vi "second_order_system_mathscript.calculate.vi"() -> ()   [LabVIEW 2015]
uses:
  <vilib>/addons/Control Design/_Model Construction/Model Typedefs.llb/CD General Elements.ctl
  <vilib>/addons/Control Design/_Model Construction/NI_LinSys_Model Typedefs.lvlib
  <vilib>/addons/Control Design/_Model Construction/Model Typedefs.llb/CD Transfer Function Model (SISO).ctl
  <vilib>/addons/Control Design/_Model Construction/Model Typedefs.llb/CD Transfer Function Model (MIMO).ctl
panel:
  in  "Step Time (s)":dbl=3.0
  in  "Gain":dbl=110000.0
  out "SysDis":T1={"properties"={"Model name"="System Model", "Input names"=["u0"], "Output names"=["y0"], "Input Delays"=[0.0], "Output Delays"=[0.0], "Sampling Time"=2e-05, "Notes"=""}, "transfer function(s)"=[[{"Numerator"=[2.19982359548343e-05, 2.1999115901172317e-05], "Denominator"=[0.9998800071997122, -1.9998777573351285, 1.0], "delay"=0.0}]]} caption="TF object" {"transfer function(s)"."delay" format="%.4f"; "transfer function(s)"."Denominator" format="%#_9e"; "transfer function(s)"."Numerator" format="%#_9e"; "properties"."Sampling Time" format="%#.6p"; "properties"."Output Delays" format="%.4f"; "properties"."Input Delays" format="%.4f"}
  in  "Ts":dbl=2e-05
  in  "NaturalFreq (r/s)":dbl=75.0
  in  "DampingRatio":dbl=0.04
  # "For the step response plot"
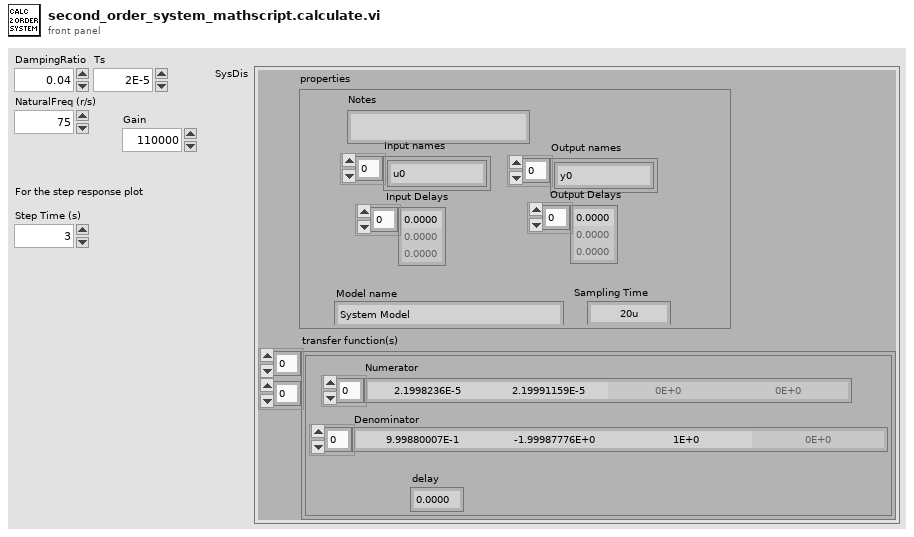
[diagram p1: front panel]
types:
  T1 = typedef "NI_LinSys_Model Typedefs.lvlib/CD Transfer Function Model (MIMO).ctl" = cluster{"properties":T2, "transfer function(s)":T3[][]}
  T2 = typedef "NI_LinSys_Model Typedefs.lvlib/CD General Elements.ctl" = cluster{"Model name":string, "Input names":string[], "Output names":string[], "Input Delays":dbl[], "Output Delays":dbl[], "Sampling Time":dbl, "Notes":string}
  T3 = typedef "NI_LinSys_Model Typedefs.lvlib/CD Transfer Function Model (SISO).ctl" = cluster{"Numerator":dbl[], "Denominator":dbl[], "delay":dbl}
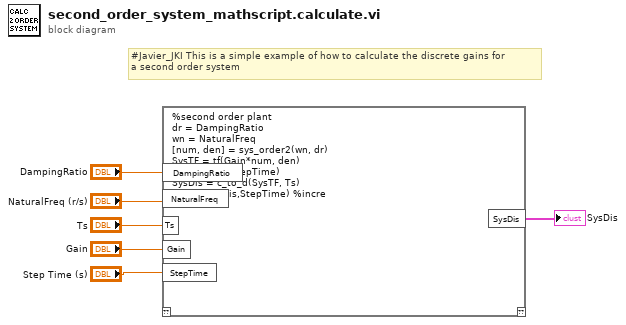
[diagram p0: block diagram]
diagram:
  # "#Javier_JKI This is a simple example of how to calculate the discrete gains for\na second order system"
  n1 = mathscript code="%second order plant\ndr = DampingRatio\nwn = NaturalFreq\n[num, den] = sys_order2(wn, dr)\nSysTF = tf(Gain*num, den)\nstep(SysTF, StepTime)\nSysDis = c_to_d(SysTF, Ts)\n%step(SysDis,StepTime) %incre"("DampingRatio"="DampingRatio", "NaturalFreq"="NaturalFreq (r/s)", "Ts"="Ts", "Gain"="Gain", "StepTime"="Step Time (s)") -> ("SysDis"=→"SysDis":T1)  [unwired: 1 in, 1 out]
